vi "WorkorderHandler_NotAReferenceConstant.vi"() -> (0 "reference":T1)   [LabVIEW 2011]
doc: "Returns a refnum whose value is Not A Refnum. You can use this refnum as an output from structures and subVIs when an error occurs."
uses:
  DataStructures/WorkorderHandler_ObjectReference.ctl
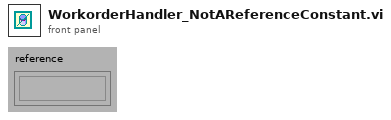
[diagram p1: front panel]
types:
  T1 = typedef "WorkorderHandler_ObjectReference.ctl" = refnum<k1>
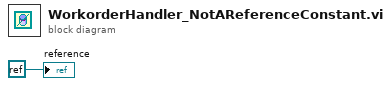
[diagram p0: block diagram]
diagram:
  "reference" <- refnum<k0> refnum
